vi "StartRecord.vi"(8 "error in (no error)":errorcluster, 10 "Label":string, 11 "NI_DAQmx(AI) in":refnum<class "NI_DAQmx(AI).lvclass">) -> (0 "error out":errorcluster, 3 "NI_DAQmx(AI) out":refnum<class "NI_DAQmx(AI).lvclass">)   [LabVIEW 2025, in "NI_DAQmx(AI).lvclass"]
uses:
  NI_DAQmx(AI).lvclass
  NI_DAQmx(AI).lvclass/NI_DAQmx(AI).ctl
  DAQ_Abstr/Task_Type/AI_Task/AI_Task/AI_Task.lvclass
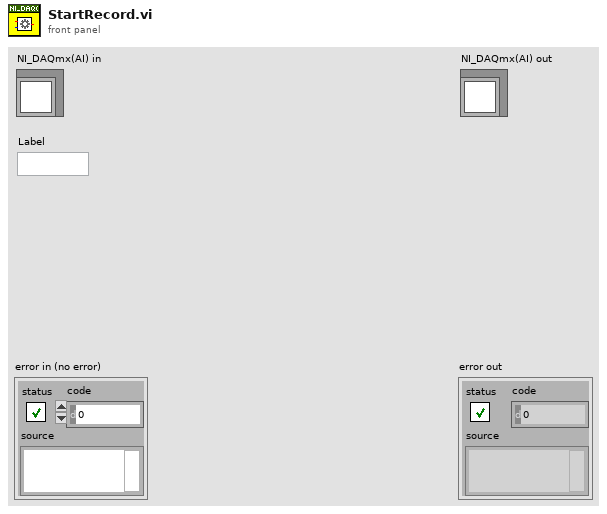
[diagram p1: front panel]
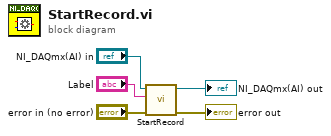
[diagram p0: block diagram]
diagram:
  n1 = call-parent "StartRecord.vi"("error in (no error)"="error in (no error)", "Label"="Label", "Task_Abstr in"="NI_DAQmx(AI) in") -> ("error out"=→"error out":errorcluster, "Task_Abstr out"=→"NI_DAQmx(AI) out":refnum<class "NI_DAQmx(AI).lvclass">)  [unwired: 7 in]
